vi "SystemNSOM.vi"() -> ()   [LabVIEW 2018]
uses:
  <vilib>/Math Plots/3D Math Plots/3D Mesh/3D Mesh XCtrl/3D Mesh.xctl
  <vilib>/Math Plots/3D Math Plots/3D Mesh/3D Mesh Datatype/3D Mesh Datatype.lvclass
  <vilib>/Math Plots/3D Math Plots/3D Mesh/3D Mesh Datatype/Public/Plot Helper (Vector).vi
panel:
  in  "thr. Ang":dbl
  out "diff Ph":dbl=9.8
  out "err R":dbl=0.1226366888094022
  in  "NUMERO DE MED.":i32=1 min=1 max=10
  in  "ControlP":T1
  in  "thr":dbl=0.1
  out "th":bool
  out "Mult inic.":dbl
  out "lock in inic.":dbl
  out "A":dbl
  in  "Nombre imagenes":string
  in  "Nombre del  Archivo":string="test_0510_01"
  in  "Atributos":T2
  in  "stop":bool
  in  "tipo":enum32{"medicion", "visualizar"}(tab)
  in  "Medir  offset":bool
  out "Z nano":dbl=15415.0
  out "Y nano":dbl=2000.0
  out "X nano":dbl=88000.0
  out "Multimetro":dbl=-0.0012043666666666666
  out "Lock in":dbl=-0.0011005000000000001
  out "X":dbl
  in  "lockinMult":T3={"Num.Lect"=3, "Delay (ms)"=1000, "usar multimetro"=TRUE, "Num. Med"=3} {"Delay (ms)" min=100; "Num.Lect" min=1}
  out "AFM":refnum<class "3D Plot Datatype.lvclass">[](xcontrol)
  in  "tipoMed":enum16{"R", "AFM", "DRL", "DRC"}(ring)
  in  "movXYZ":T4={"Inicio x"=0.0, "Inicio y"=0.0, "fin x"=88000.0, "fin y "=2000.0, "paso"=2000.0, "selector"=FALSE}
  out "Lockin":refnum<class "3D Plot Datatype.lvclass">[](xcontrol)
  in  "Inicio":bool
  out "Y":dbl
  out "Z":dbl
  out "multimetro":refnum<class "3D Plot Datatype.lvclass">[](xcontrol)
  in  "Distancia de medicion":dbl=9.0
  out "Amplitud":dbl[](graph)=[0.0001737, 0.0001907, 0.0001951, 0.0001957, 0.0001958, 0.0001961, 0.0001961, 0.000196, 0.0001957, 0.0001957, 0.000196, 0.000196, 0.0001958, 0.000196, 0.000196, 0.0001958, 0.0001957, 0.0001957, 0.000196, 0.0001963, 0.0001963, 0.0001966, 0.0001966, 0.0001963, 0.0001965, 0.0001967, 0.0001966, 0.0001966, 0.0001966, 0.0001968, 0.000197, 0.000197, 0.000197, 0.0001968, 0.0001967, 0.0001967, 0.0001966, 0.0001966, 0.0001962, 0.000196, 0.0001961, 0.0001963, 0.0001962, 0.0001962, 0.0001962, 0.0001963, 0.0001965, 0.0001963, 0.0001962, 0.0001961, 0.0001958, 0.0001958, 0.0001958, 0.0001957, 0.0001955, 0.0001955, 0.000196, 0.0001961, 0.0001958, 0.0001956, 0.000196, 0.0001958, 0.0001958, 0.000196, 0.0001958, 0.000196, 0.0001958, 0.0001958, 0.0001958, 0.0001956, 0.0001952, 0.0001952, 0.0001956, 0.0001956, 0.0001957, 0.0001956, 0.0001955, 0.0001958, 0.0001958, 0.0001961, 0.0001962, 0.0001962, 0.0001963, 0.0001966, 0.0001965, 0.0001966, 0.0001966, 0.0001968, 0.0001968, 0.0001966, 0.0001961, 0.0001962, 0.0001965, 0.0001967, 0.0001963, 0.0001961, 0.0001958, 0.0001963, 0.0001966, 0.0001965, 0.0001963, 0.0001961, 0.0001961, 0.0001966, 0.0001968, 0.0001967, 0.0001963, 0.0001961, 0.0001961, 0.0001961, 0.0001958, 0.0001957, 0.0001956, 0.0001957, 0.0001955, 0.0001956, 0.0001958, 0.0001952, 0.0001958, 0.0001958, 0.0001955, 0.0001955, 0.0001955, 0.0001961, 0.0001963, 0.0001965, 0.0001962, 0.000196, 0.0001963, 0.0001966, 0.0001966, 0.0001966, 0.0001963, 0.0001963, 0.0001966, 0.0001966, 0.0001966, 0.0001965, 0.0001963, 0.0001966, 0.0001967, 0.0001968, 0.0001967, 0.0001966, 0.0001966, 0.0001967, 0.0001966, 0.0001965, 0.0001963, 0.0001967, 0.0001963, 0.0001961, 0.0001956, 0.0001956, 0.0001956, 0.0001956, 0.0001955, 0.0001952, 0.0001952, 0.0001952, 0.0001955, 0.0001957, 0.0001956, 0.0001956, 0.0001956, 0.0001957, 0.0001958, 0.0001958, 0.0001956, 0.0001955, 0.0001956, 0.0001958, 0.0001957, 0.0001956, 0.0001956, 0.0001956, 0.0001958, 0.0001957, 0.0001955, 0.0001956, 0.000196, 0.0001958, 0.0001961, 0.000196, 0.000196, 0.0001958, 0.0001965, 0.0001963, 0.0001966, 0.0001965, 0.0001965, 0.0001965, 0.0001963, 0.0001963, 0.0001961, 0.0001961, 0.0001966, 0.0001966, 0.0001966, 0.0001965, 0.0001958, 0.000196, 0.0001962, 0.0001962, 0.0001965, 0.0001962, 0.0001963, 0.0001965, 0.0001963, 0.0001965, 0.0001961, 0.0001961, 0.0001961, 0.0001961, 0.0001962, 0.000196, 0.0001956, 0.0001961, 0.0001961, 0.0001958, 0.0001956, 0.0001953, 0.0001953, 0.0001956, 0.0001956, 0.0001953, 0.0001953, 0.0001955, 0.0001956, 0.0001955, 0.0001953, 0.0001952, 0.0001952, 0.0001957, 0.0001958, 0.0001958, 0.0001958, 0.0001958, 0.0001958, 0.0001958, 0.0001956, 0.0001955, 0.0001957, 0.000196, 0.0001961, 0.0001958, 0.0001957, 0.0001957, 0.0001958, 0.0001961, 0.0001961, 0.0001961, 0.0001958, 0.0001958, 0.0001961, 0.0001965, 0.0001963, 0.0001965, 0.0001965, 0.0001965, 0.0001962, 0.0001963, 0.0001963, 0.0001961, 0.0001961, 0.0001958, 0.0001958, 0.000196, 0.0001958, 0.0001955, 0.0001956, 0.0001958, 0.0001956, 0.0001955, 0.0001957, 0.0001958, 0.0001958, 0.0001958, 0.0001956, 0.0001953, 0.0001953, 0.0001955, 0.0001953, 0.000195, 0.0001947, 0.0001948, 0.0001951, 0.0001951, 0.000195, 0.0001946, 0.0001948, 0.0001948, 0.0001952, 0.000195, 0.000195, 0.0001953, 0.0001956, 0.0001956, 0.0001958, 0.0001958, 0.0001961, 0.0001961, 0.000196, 0.0001958, 0.000196, 0.0001962, 0.0001965, 0.0001961, 0.000196, 0.0001955, 0.0001975, 0.0001981, 0.0001973, 0.0001966, 0.0001957, 0.0001953, 0.0001948, 0.0001946, 0.0001942, 0.0001933, 0.0001905, 0.0001845, 0.0001812, 0.0001717]
  out "Fase":dbl[](graph)=[1.35, -1.7, -2.3, -2.4, -2.4, -2.4, -2.35, -2.4, -2.4, -2.45, -2.45, -2.45, -2.45, -2.4, -2.4, -2.4, -2.4, -2.4, -2.45, -2.4, -2.4, -2.4, -2.4, -2.4, -2.45, -2.45, -2.45, -2.45, -2.5, -2.45, -2.4, -2.45, -2.4, -2.4, -2.4, -2.4, -2.45, -2.4, -2.45, -2.5, -2.5, -2.5, -2.45, -2.45, -2.5, -2.5, -2.45, -2.45, -2.45, -2.45, -2.45, -2.45, -2.45, -2.45, -2.5, -2.5, -2.45, -2.45, -2.45, -2.5, -2.5, -2.45, -2.4, -2.4, -2.4, -2.4, -2.45, -2.45, -2.45, -2.45, -2.5, -2.45, -2.45, -2.45, -2.4, -2.45, -2.5, -2.45, -2.5, -2.5, -2.55, -2.45, -2.45, -2.45, -2.45, -2.45, -2.45, -2.45, -2.45, -2.4, -2.45, -2.45, -2.45, -2.45, -2.45, -2.55, -2.6, -2.5, -2.5, -2.45, -2.5, -2.55, -2.6, -2.55, -2.45, -2.45, -2.45, -2.5, -2.5, -2.55, -2.45, -2.45, -2.45, -2.55, -2.5, -2.45, -2.55, -2.55, -2.5, -2.45, -2.5, -2.5, -2.5, -2.5, -2.45, -2.45, -2.45, -2.55, -2.55, -2.5, -2.5, -2.5, -2.55, -2.55, -2.5, -2.5, -2.5, -2.55, -2.55, -2.55, -2.55, -2.55, -2.55, -2.45, -2.55, -2.5, -2.5, -2.45, -2.5, -2.55, -2.5, -2.5, -2.55, -2.55, -2.55, -2.55, -2.55, -2.6, -2.65, -2.6, -2.55, -2.45, -2.45, -2.5, -2.55, -2.55, -2.55, -2.55, -2.5, -2.6, -2.55, -2.65, -2.55, -2.55, -2.55, -2.5, -2.6, -2.55, -2.55, -2.6, -2.6, -2.6, -2.55, -2.6, -2.6, -2.6, -2.65, -2.6, -2.55, -2.55, -2.55, -2.55, -2.5, -2.55, -2.6, -2.65, -2.7, -2.65, -2.65, -2.65, -2.7, -2.7, -2.6, -2.65, -2.65, -2.65, -2.6, -2.6, -2.55, -2.65, -2.65, -2.6, -2.6, -2.55, -2.55, -2.55, -2.6, -2.6, -2.55, -2.6, -2.6, -2.65, -2.6, -2.65, -2.55, -2.6, -2.55, -2.55, -2.6, -2.6, -2.6, -2.65, -2.6, -2.6, -2.6, -2.6, -2.65, -2.6, -2.6, -2.5, -2.55, -2.6, -2.7, -2.65, -2.6, -2.65, -2.7, -2.7, -2.7, -2.6, -2.55, -2.55, -2.6, -2.65, -2.6, -2.55, -2.6, -2.7, -2.7, -2.65, -2.6, -2.6, -2.6, -2.6, -2.55, -2.6, -2.65, -2.6, -2.65, -2.55, -2.5, -2.5, -2.55, -2.55, -2.6, -2.6, -2.65, -2.65, -2.6, -2.65, -2.65, -2.65, -2.65, -2.7, -2.65, -2.6, -2.6, -2.55, -2.55, -2.55, -2.65, -2.6, -2.65, -2.6, -2.65, -2.65, -2.65, -2.65, -2.65, -2.65, -2.6, -2.6, -2.6, -2.65, -2.65, -2.7, -2.65, -2.6, -2.55, 1.85, 14.25, 17.75, 19.65, 21.45, 22.75, 23.6, 24.45, 25.2, 25.05, 23.35, 15.35, 3.05, 0.4, 7.4]
  in  "Tipo Stop":enum16{"Amplitud", "Fase"}(ring)
  in  "nanoREc":bool
  in  "Ajuste":bool
  in  "camara":bool
  # "Lock in"
  # "Multimetro"
  # "Parámetros de barrido"
  # "micras"
  # "nanometros"
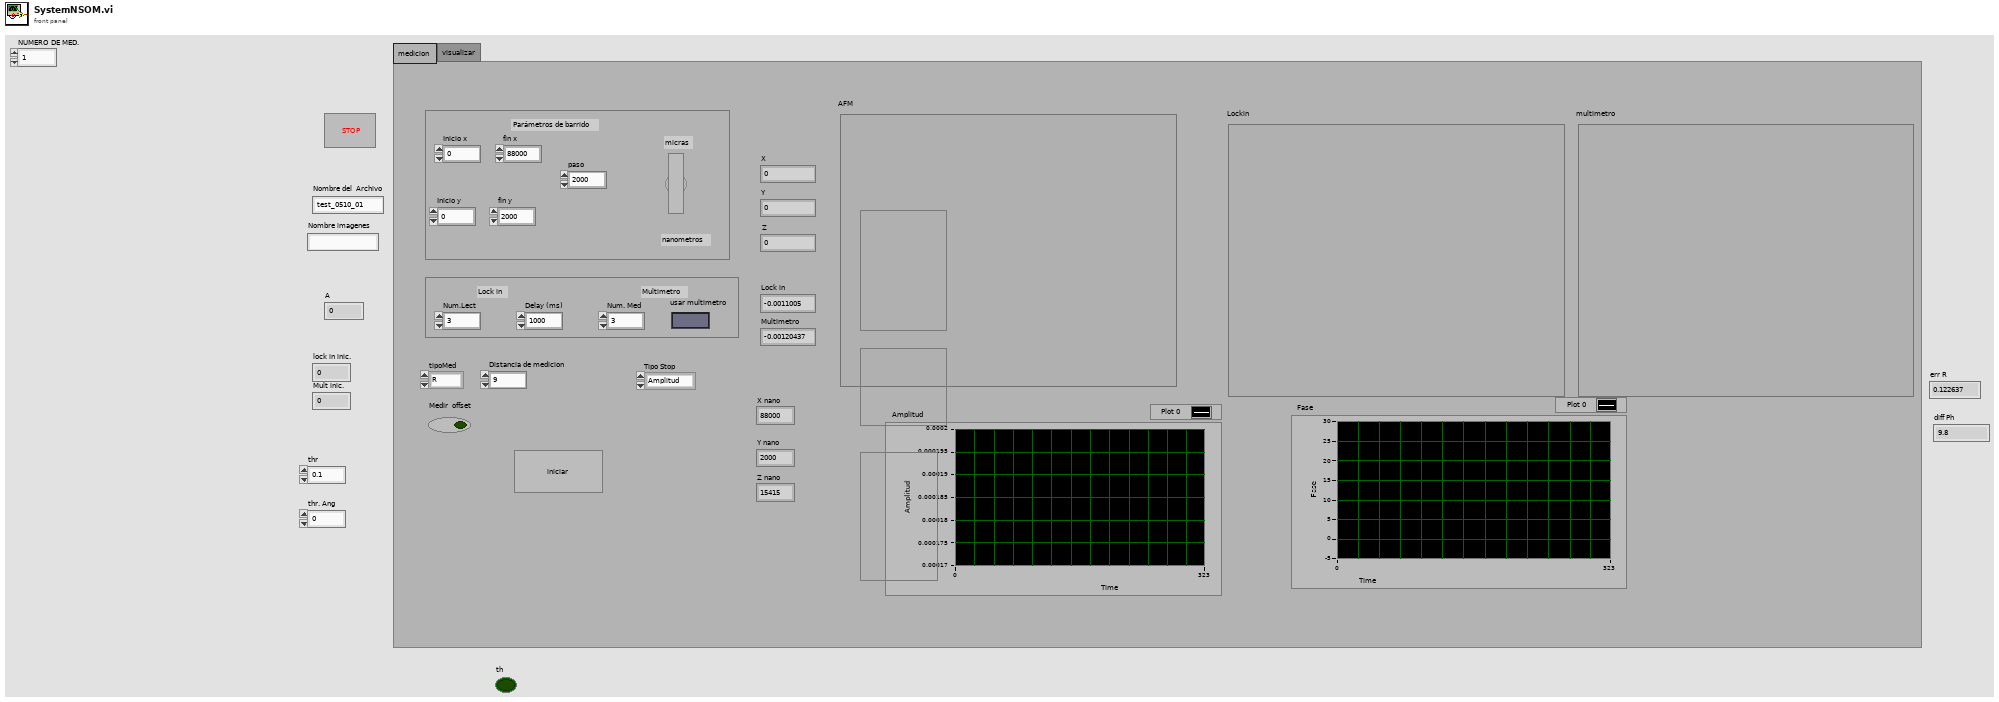
[diagram p1: front panel]
types:
  T1 = cluster{"posicion":dbl, "Amplitud":dbl[], "Fase":dbl[], "Err A":dbl, "Dif Ph":dbl, "Inic. A":dbl, "Inic. Ph":dbl}
  T2 = cluster{"Inicio X":dbl, "Inicio Y":dbl, "fin X ":dbl, "paso":dbl, "fin Y ":dbl, "Unidades":string, "Tipo":string}
  T3 = cluster{"Num.Lect":i32, "Delay (ms)":i32, "usar multimetro":bool, "Num. Med":i32}
  T4 = cluster{"Inicio x":dbl, "Inicio y":dbl, "fin x":dbl, "fin y ":dbl, "paso":dbl, "selector":bool}
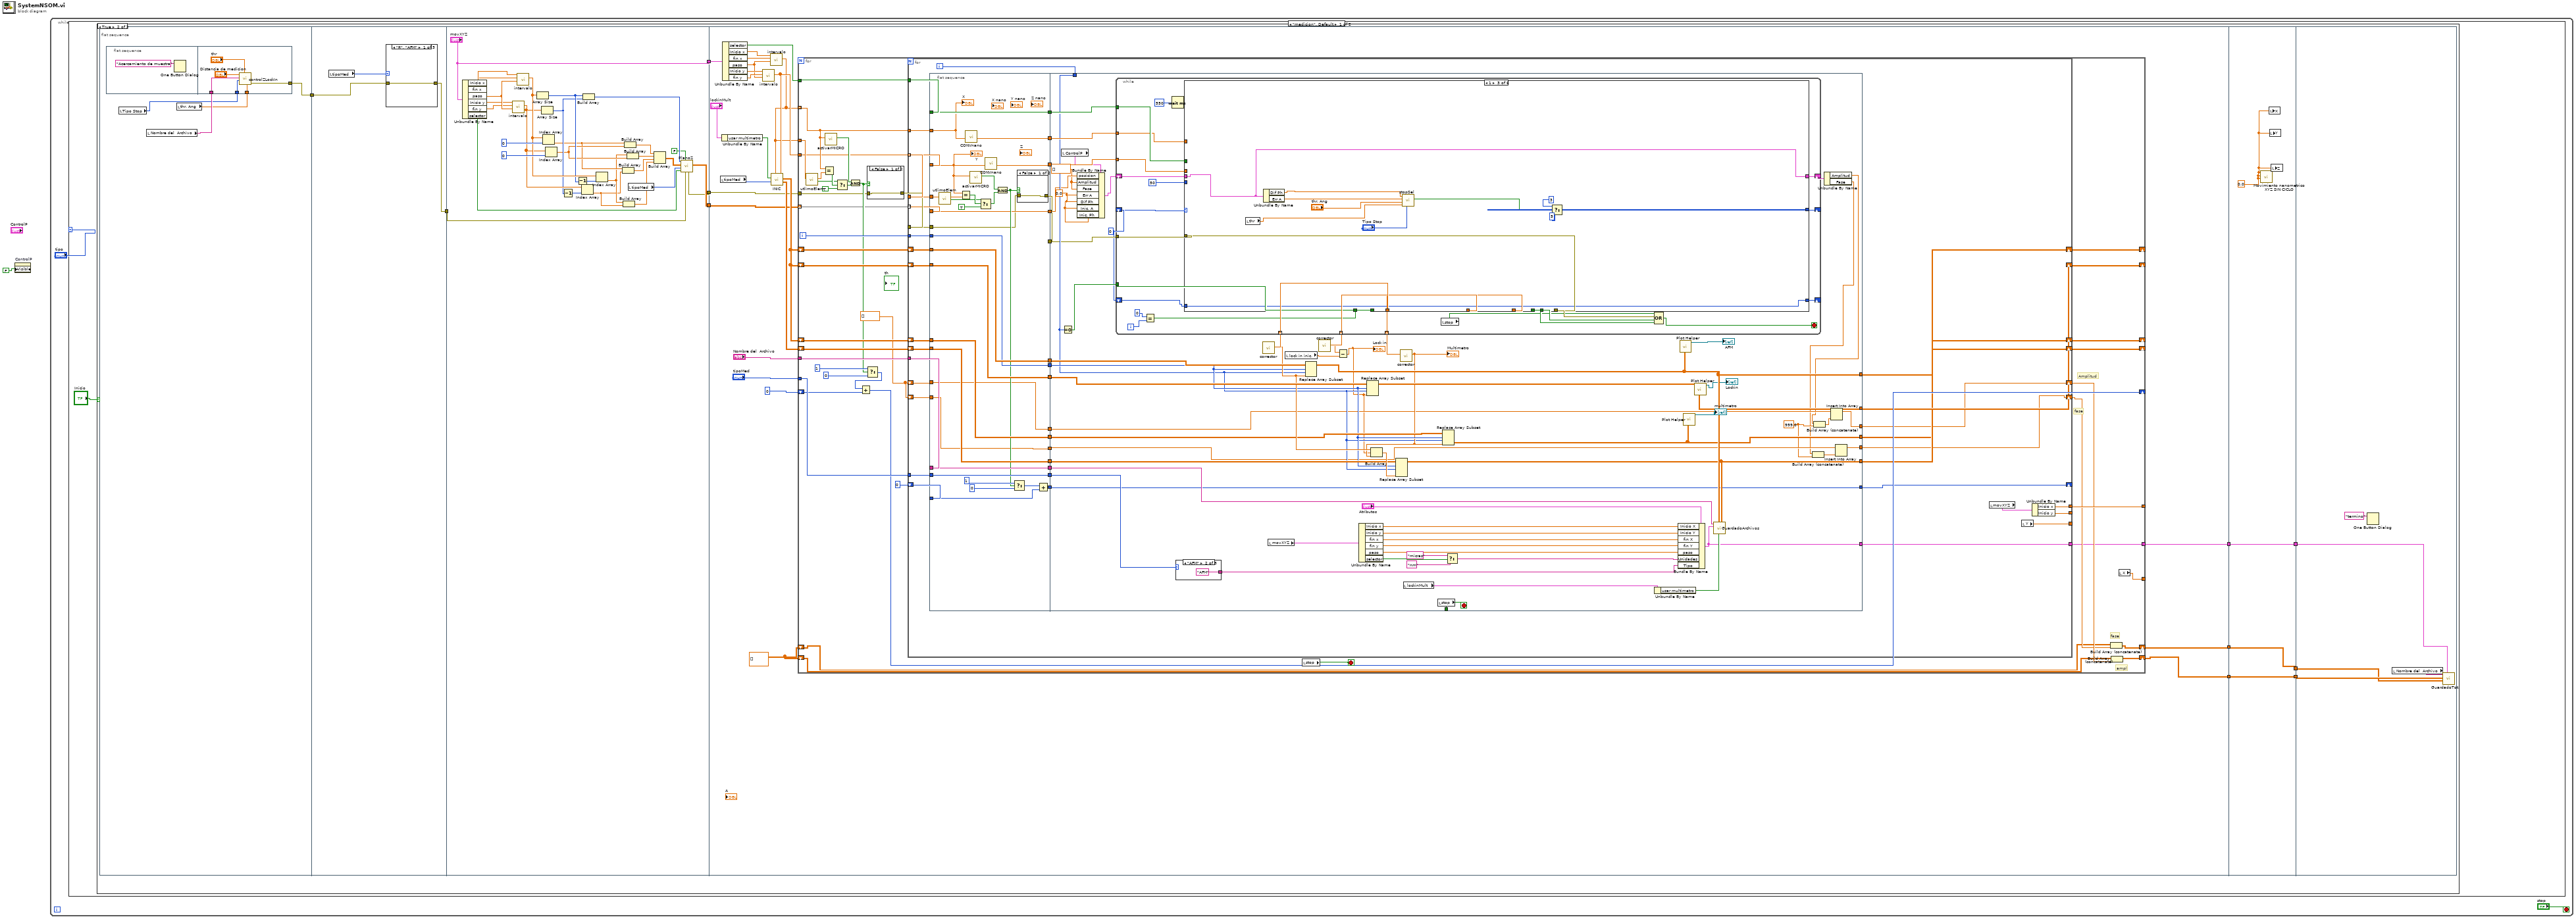
[diagram p0: block diagram]
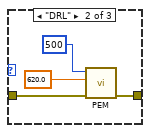
[diagram p3: hidden frame]
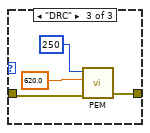
[diagram p4: hidden frame]
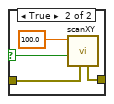
[diagram p5: hidden frame]
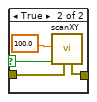
[diagram p6: hidden frame]
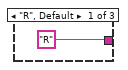
[diagram p7: hidden frame]
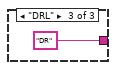
[diagram p8: hidden frame]
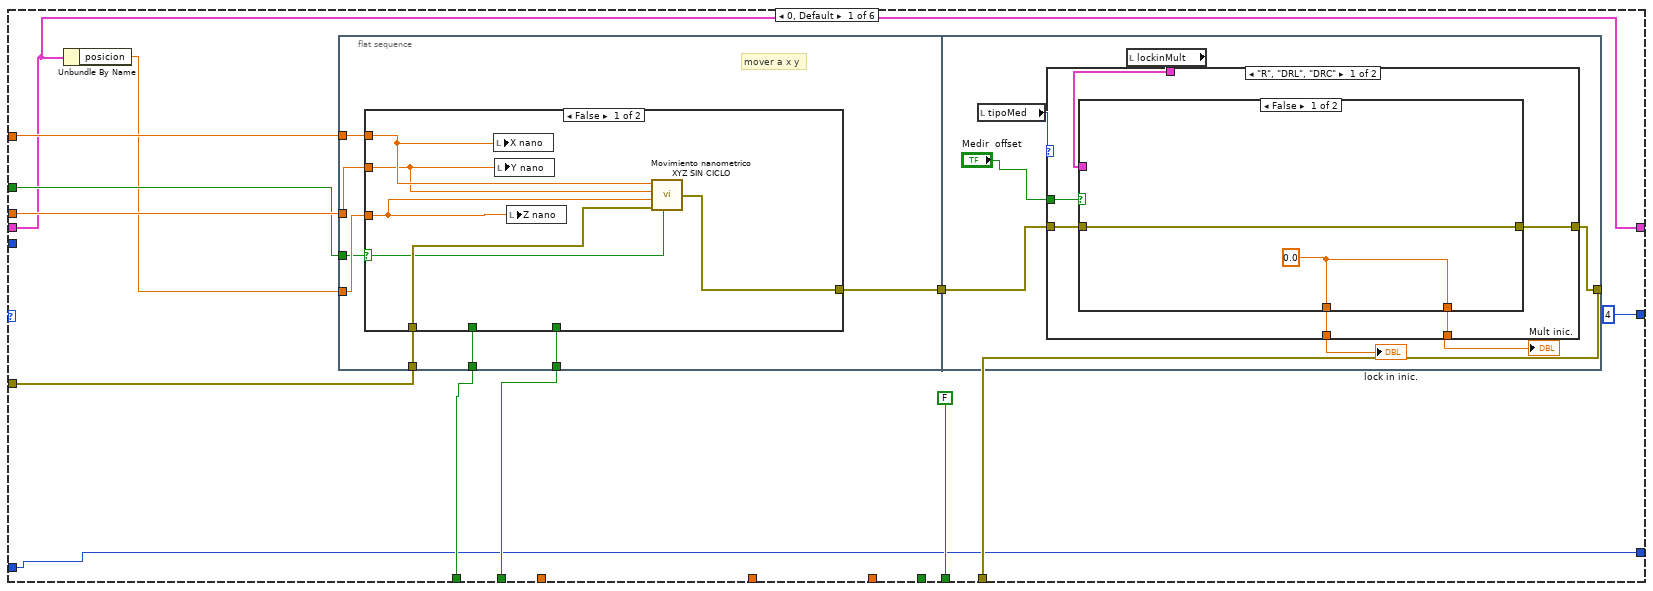
[diagram p9: hidden frame]
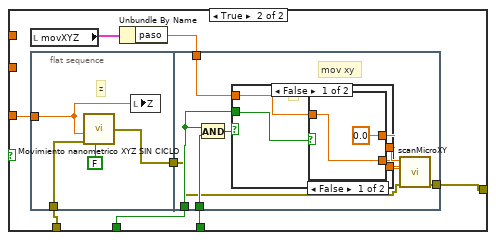
[diagram p10: hidden frame]
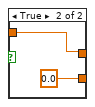
[diagram p11: hidden frame]
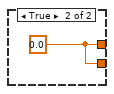
[diagram p12: hidden frame]
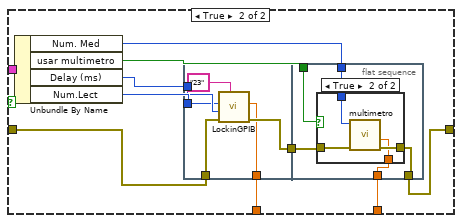
[diagram p13: hidden frame]
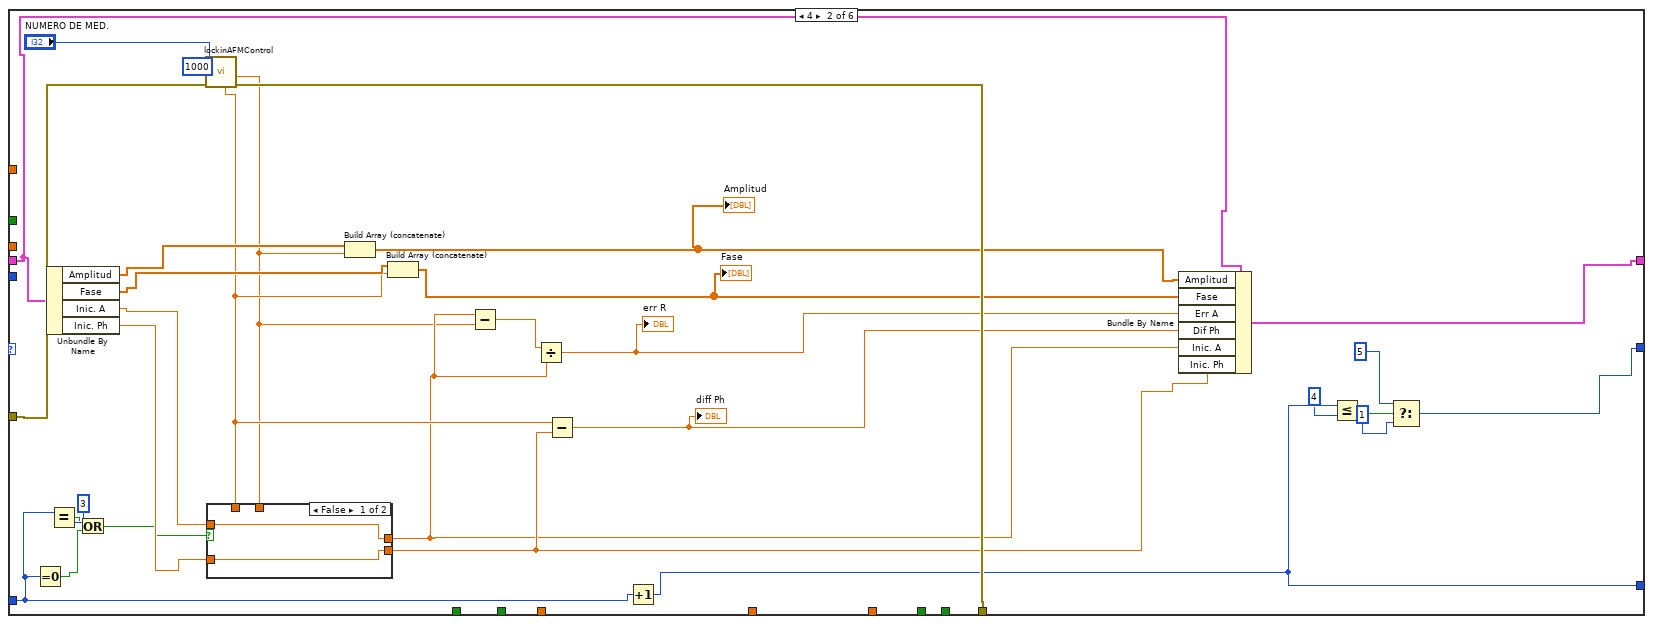
[diagram p16: hidden frame]
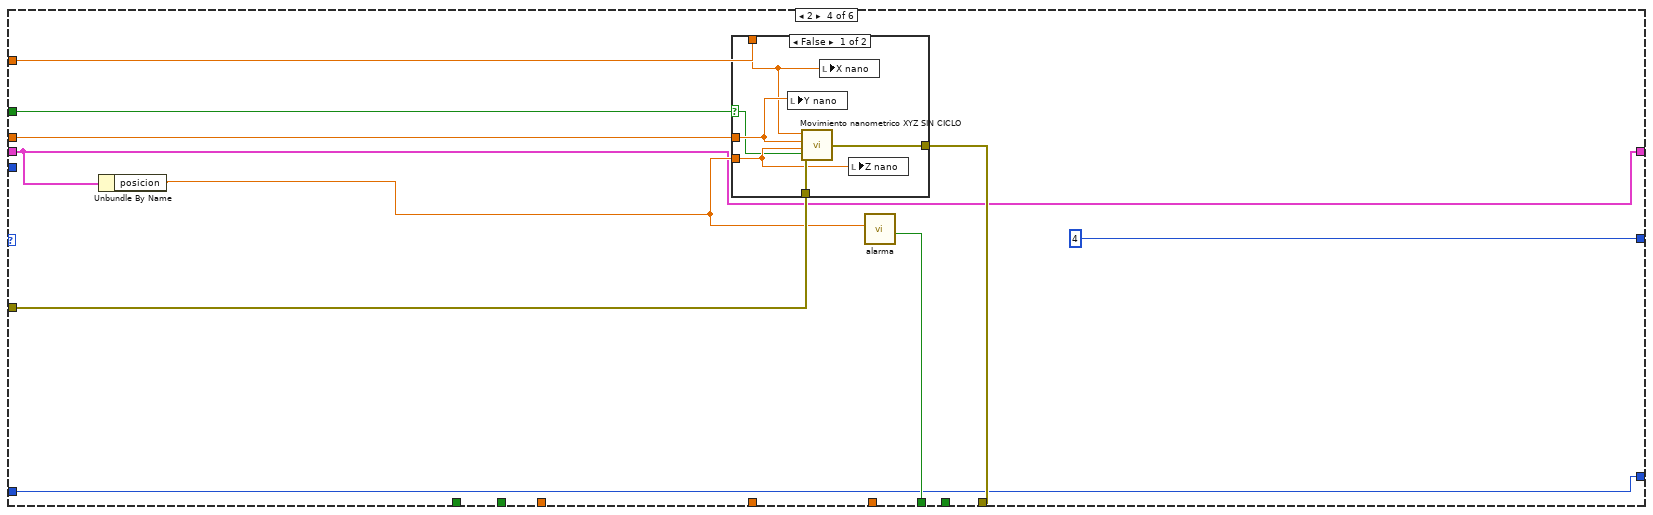
[diagram p18: hidden frame]
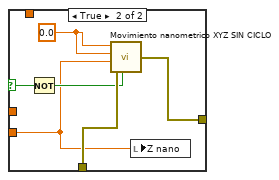
[diagram p19: hidden frame]
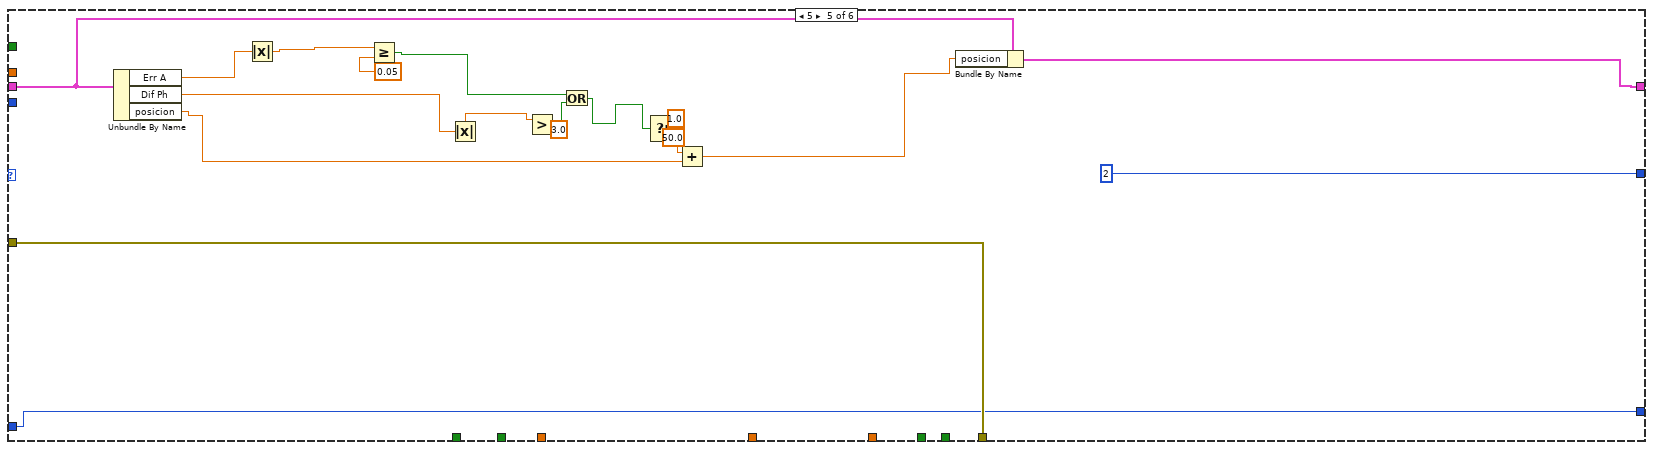
[diagram p20: hidden frame]
diagram:
  n1 = property on="ControlP" class="Clust (strict)"("Visible"=FALSE) -> ()  [unwired: 2 in, 2 out]
  n2 = while {
    stop <- "stop" stop-if-true
    n3 = case shown="\"medicion\", Default" "tipo" {
      frame "medicion", Default {
        n4 = case shown="True" "Inicio" {
          frame False {
          }
          frame True {
            n5 = flat-sequence {
              tunnel: [w19] -> w11
              tunnel: [w28] -> w12
              tunnel: w11 -> [w27]
              tunnel: ["movXYZ"] -> w15
              tunnel: [w44] -> w14
              tunnel: [w42] -> w13
              tunnel: w12 -> [w41]
              tunnel: w15 -> [w76]
              tunnel: w14 -> [w75]
              tunnel: w13 -> [w72]
              tunnel: [w73] -> w10
              tunnel: [w70] -> w7
              tunnel: [w69] -> w5
              tunnel: w10 -> [w571]
              tunnel: [w571] -> w9
              tunnel: [w570] -> w8
              tunnel: w7 -> [w570]
              tunnel: [w569] -> w6
              tunnel: w5 -> [w569]
              tunnel: w9 -> [w576]
              tunnel: w8 -> [w575]
              tunnel: w6 -> [w573]
              frame #0 {
                n6 = flat-sequence {
                  tunnel: [w25] -> w19
                  tunnel: w18 -> [w24]
                  tunnel: w17 -> [w22]
                  tunnel: w16 -> [w21]
                  frame #0 {
                    n7 = One Button Dialog(message="Acercamiento de muestra") -> ()  [unwired: 1 in, 1 out]
                  }
                  frame #1 {
                    n8 = call "controlZLockIn.vi"("thrAng"=w22, "thr"="thr", "Tipo"=w21, "name"=w24, "Distancia de medicion"="Distancia de medicion") -> ("error out"=w25:errorcluster)  [unwired: 3 in, 3 out]
                  }
                }
                n9 = local read "Tipo Stop"() -> (w16:enum16{"Amplitud", "Fase"})
                n10 = local read "Nombre del  Archivo"() -> (w18:string)
                n11 = local read "thr. Ang"() -> (w17:dbl)
              }
              frame #1 {
                n12 = local read "tipoMed"() -> (w29:enum16{"R", "AFM", "DRL", "DRC"})
                n13 = case shown="\"R\", \"AFM\"" w29 {
                  tunnel: [w30 w32 w36] -> w28
                  tunnel: w27 -> [w30 w31 w35]
                  frame "R", "AFM" {
                  }
                  frame "DRL" {
                    n14 = call "PEM.vi"("error in (no error)"=w31, "Longitud de Onda"=620.0, "Retardo"=500) -> ("error out"=w32:errorcluster)  [unwired: 6 in, 2 out]
                  }
                  frame "DRC" {
                    n15 = call "PEM.vi"("error in (no error)"=w35, "Longitud de Onda"=620.0, "Retardo"=250) -> ("error out"=w36:errorcluster)  [unwired: 6 in, 2 out]
                  }
                }
              }
              frame #2 {
                n16 = Unbundle By Name("movXYZ") -> ("Inicio x"=w67:dbl, "fin x"=w66:dbl, "paso"=w65:dbl, "Inicio y"=w64:dbl, "fin y"=w63:dbl, "selector"=w40:bool)
                n17 = call "intervalo.vi"("incremento"=w65, "fin"=w63, "inicio"=w64) -> ("Array"=w58:dbl[])  [unwired: 8 in]
                n18 = call "intervalo.vi"("incremento"=w65, "fin"=w66, "inicio"=w67) -> ("Array"=w59:dbl[])  [unwired: 8 in]
                n19 = Array Size(array=w59) -> (size(s)=w57:i32)
                n20 = Array Size(array=w58) -> (size(s)=w55:i32)
                n21 = Index Array(array=w59, index=0) -> (element=w52:dbl)
                n22 = Index Array(array=w58, index=0) -> (element=w53:dbl)
                n23 = Decrement(x=w55) -> (x-1=w54:i32)
                n24 = Decrement(x=w57) -> (x-1=w56:i32)
                n25 = Index Array(array=w58, index=w54) -> (element=w50:dbl)
                n26 = Build Array(w57, w55) -> (w62:i32[])
                n27 = Index Array(array=w59, index=w56) -> (element=w51:dbl)
                n28 = Build Array(w52, w50) -> (w47:dbl[])
                n29 = Build Array(w51, w50) -> (w46:dbl[])
                n30 = Build Array(w52, w53) -> (w49:dbl[])
                n31 = Build Array(w51, w53) -> (w48:dbl[])
                n32 = local read "tipoMed"() -> (w43:enum16{"R", "AFM", "DRL", "DRC"})
                n33 = Build Array(w49, w48, w47, w46) -> (w45:dbl[][])
                n34 = call "PlanoZ.vi"("error in (no error)"=w41, "Pendiente"=FALSE, "tipo"=w40, "tipoMed"=w43, "MedicionesPuntos"=w45, "Tamaños"=w62) -> ("PosZ"=w44:dbl[][], "error out"=w42:errorcluster)  [unwired: 4 in]
              }
              frame #3 {
                w71 = dbl[][] []
                n35 = local read "tipoMed"() -> (w78:enum16{"R", "AFM", "DRL", "DRC"})
                n36 = Unbundle By Name("lockinMult") -> ("usar multimetro"=w81:bool)
                n37 = Unbundle By Name(w76) -> ("selector"=w86:bool, "Inicio x"=w90:dbl, "fin x"=w91:dbl, "paso"=w87:dbl, "Inicio y"=w89:dbl, "fin y"=w88:dbl)
                n38 = call "intervalo.vi"("incremento"=w87, "fin"=w88, "inicio"=w89) -> ("Array"=w85:dbl[])  [unwired: 8 in]
                n39 = call "intervalo.vi"("incremento"=w87, "fin"=w91, "inicio"=w90) -> ("Array"=w74:dbl[])  [unwired: 8 in]
                n40 = call "INIC.vi"("ArrY"=w85, "ArrX"=w74, "tipoMed"=w78, "mutl"=w81) -> ("ArrSal4"=w80:dbl[][][], "ArrSAL"=w79:dbl[][])  [unwired: 6 in]
                n41 = for {
                  tunnel: w74 -> [w109] mode=indexing
                  tunnel: w85 -> [w107]
                  tunnel: w86 -> [w133]
                  shift-right: [w131] -> _
                  shift-left: w79 -> [w132]
                  tunnel: "tipoMed" -> [w129]
                  tunnel: "Nombre del  Archivo" -> [w128]
                  shift-right: [w126] -> _
                  shift-left: w79 -> [w127]
                  shift-right: [w124] -> _
                  shift-left: w80 -> [w125]
                  shift-right: [w121] -> _
                  shift-left: w79 -> [w122]
                  shift-right: [w110] -> _
                  shift-left: 0 -> [w111]
                  tunnel: w74 -> [w108]
                  tunnel: w75 -> [w104] mode=indexing
                  tunnel: w72 -> [w102]
                  tunnel: [w101] -> _
                  tunnel: [w100] -> _
                  shift-right: [w99] -> w73
                  shift-left: w71 -> [w97]
                  shift-right: [w95] -> w70
                  shift-left: w71 -> [w93]
                  tunnel: [w92] -> w69
                  i -> [w130]
                  stop <- w123 stop-if-true
                  w96 = dbl[] []
                  # "ampl"
                  # "fase"
                  # "fase"
                  # "Amplitud"
                  n42 = call "utlimoElem.vi"("Elementos"=w108) -> ("x = 0?"=w118:bool, "element"=w120:dbl)  [unwired: 9 in]
                  n43 = Equal?(x=w109, y=w120) -> (x = y?=w119:bool)
                  n44 = call "activarMICRO.vi"("valor"=w109) -> ("Indicador"=w115:bool)  [unwired: 10 in]
                  n45 = Select(t=w118, s=w119, f=TRUE) -> (s? t:f=w116:bool)
                  n46 = And(x=w115, y=w116) -> (x .and. y?=w105:bool)
                  n47 = case shown="False" w105 {
                    selector: w105 -> [_ w137]
                    tunnel: [w134 w136] -> w103
                    tunnel: w102 -> [w134 w135]
                    frame False {
                    }
                    frame True {
                      n48 = call "scanXY.vi"("Error In"=w135, "Activar movimiento en X"=w137, "Micras en X"=100.0) -> ("Error Out"=w136:errorcluster)  [unwired: 8 in]
                    }
                  }
                  n49 = Select(t=1, s=w105, f=0) -> (s? t:f=w114:i32)
                  n50 = Add(x=w114, y=w111) -> (x+y=w110:i32)
                  n51 = for {
                    tunnel: w109 -> [w181]
                    tunnel: w107 -> [w182] mode=indexing
                    tunnel: w133 -> [w183]
                    shift-right: [w179] -> w131
                    shift-left: w132 -> [w180]
                    tunnel: w130 -> [w170]
                    tunnel: w129 -> [w178]
                    tunnel: w128 -> [w177]
                    shift-right: [w174] -> w126
                    shift-left: w127 -> [w176]
                    shift-right: [w173] -> w124
                    shift-left: w125 -> [w175]
                    shift-right: [w168] -> w121
                    shift-left: w122 -> [w171]
                    tunnel: w107 -> [w167]
                    shift-right: [w165] -> _
                    shift-left: 0 -> [w166]
                    tunnel: w104 -> [w164] mode=indexing
                    tunnel: w103 -> [w163]
                    tunnel: [w162] -> _
                    tunnel: [w160] -> w101
                    tunnel: [w159] -> _
                    shift-right: [w157] -> w98
                    shift-left: w96 -> [w158]
                    shift-right: [w140] -> w94
                    shift-left: w96 -> [w141]
                    tunnel: [w139] -> w92
                    i -> [w169]
                    stop <- w172 stop-if-true
                    n52 = flat-sequence {
                      tunnel: w170 -> [w206]
                      tunnel: w171 -> [w207]
                      tunnel: w175 -> [w208]
                      tunnel: w176 -> [w209]
                      tunnel: w177 -> [w210]
                      tunnel: w178 -> [w211]
                      tunnel: w180 -> [w212]
                      tunnel: w181 -> [w193]
                      tunnel: w182 -> [w191]
                      tunnel: w183 -> [w213]
                      tunnel: [w213] -> w156
                      tunnel: [w190] -> w155
                      tunnel: [w192] -> w154
                      tunnel: [w212] -> w153
                      tunnel: [w211] -> w152
                      tunnel: [w210] -> w151
                      tunnel: [w209] -> w150
                      tunnel: [w208] -> w149
                      tunnel: [w207] -> w148
                      tunnel: [w206] -> w147
                      tunnel: w167 -> [w201]
                      tunnel: w166 -> [w195]
                      tunnel: [w194] -> w146
                      tunnel: [w188] -> w145
                      tunnel: w164 -> [w188]
                      tunnel: [w187] -> w144
                      tunnel: w163 -> [w186]
                      tunnel: w158 -> [w185]
                      tunnel: [w185] -> w143
                      tunnel: [w184] -> w142
                      tunnel: w141 -> [w184]
                      tunnel: [w271] -> w179
                      tunnel: [w255] -> w174
                      tunnel: [w254] -> w173
                      tunnel: [w251] -> w172
                      tunnel: w169 -> [w241]
                      tunnel: [w244] -> w168
                      tunnel: w156 -> [w280]
                      tunnel: w155 -> [w279]
                      tunnel: w154 -> [w278]
                      tunnel: w153 -> [w276]
                      tunnel: w152 -> [w262]
                      tunnel: w151 -> [w260]
                      tunnel: w150 -> [w258]
                      tunnel: w149 -> [w256]
                      tunnel: w148 -> [w247]
                      tunnel: w147 -> [w246]
                      tunnel: [w242] -> w165
                      tunnel: w146 -> [w242]
                      tunnel: w145 -> [w232]
                      tunnel: w144 -> [w240]
                      tunnel: w143 -> [w239]
                      tunnel: [w238] -> w157
                      tunnel: w142 -> [w226]
                      tunnel: [w225] -> w140
                      tunnel: [w224] -> w139
                      frame #0 {
                        n53 = call "utlimoElem.vi"("Elementos"=w201) -> ("x = 0?"=w200:bool, "element"=w205:dbl)  [unwired: 9 in]
                        n54 = Equal?(x=w191, y=w205) -> (x = y?=w204:bool)
                        n55 = call "CONVnano.vi"("vAL"=w193) -> ("NANO"=w192:dbl)  [unwired: 10 in]
                        n56 = call "activarMICRO.vi"("valor"=w191) -> ("Indicador"=w199:bool)  [unwired: 10 in]
                        n57 = Select(t=w200, s=w204, f=TRUE) -> (s? t:f=w202:bool)
                        n58 = call "CONVnano.vi"("vAL"=w191) -> ("NANO"=w190:dbl)  [unwired: 10 in]
                        n59 = And(x=w199, y=w202) -> (x .and. y?=w189:bool)
                        n60 = Select(t=1, s=w189, f=0) -> (s? t:f=w198:i32)
                        n61 = case shown="False" w189 {
                          selector: w189 -> [_ w217]
                          tunnel: [w214 w216] -> w187
                          tunnel: w186 -> [w214 w215]
                          frame False {
                          }
                          frame True {
                            n62 = call "scanXY.vi"("Error In"=w215, "Activar movimiento en Y"=w217, "Micras en Y"=100.0) -> ("Error Out"=w216:errorcluster)  [unwired: 8 in]
                          }
                        }
                        n63 = Add(x=w198, y=w195) -> (x+y=w194:i32)
                        "X" <- w193
                        "Y" <- w191
                      }
                      frame #1 {
                        w221 = 999.0
                        w229 = 0.0
                        w231 = dbl[] []
                        w228 = 0
                        n64 = local read "ControlP"() -> (w233:T1)
                        n65 = Equal To 0?(x=w241) -> (x = 0?=w234:bool)
                        n66 = Bundle By Name(cluster=w233, "posicion"=w232, "Amplitud"=w231, "Fase"=w231, "Err A"=w229, "Dif Ph"=w229, "Inic. A"=w229, "Inic. Ph"=w229) -> (w230:T1)
                        n67 = while {
                          shift-right: [w306] -> _
                          shift-left: w228 -> [w307]
                          tunnel: w280 -> [w305]
                          tunnel: w278 -> [w297]
                          tunnel: w279 -> [w296]
                          tunnel: [w304] -> w277 mode=indexing
                          tunnel: [w300] -> w259 mode=indexing
                          tunnel: [w295] -> w248 mode=indexing
                          tunnel: w234 -> [w291]
                          tunnel: w240 -> [w292]
                          shift-right: [w286] -> w227
                          shift-left: w230 -> [w287]
                          shift-right: [w284] -> _
                          shift-left: w228 -> [w285]
                          i -> [w290]
                          stop <- w303 stop-if-true
                          n68 = Equal?(x=0, y=w290) -> (x = y?=w289:bool)
                          n69 = Wait (ms)(milliseconds to wait=u32 550) -> ()  [unwired: 1 out]
                          n70 = case shown="1" w307 {
                            tunnel: [4 w410 w450 4 2 0] -> w306
                            tunnel: w305 -> [w314 _ _ w455 _ _]
                            tunnel: w292 -> [w320 w435 w449 w461 w491 w504]
                            tunnel: [w319 w432 w449 w459 w491 w503] -> w302
                            tunnel: w297 -> [w316 _ _ w456 _ _]
                            tunnel: w296 -> [w315 _ _ w457 _ _]
                            tunnel: [_ _ _ _ _ w507] -> w304
                            tunnel: [FALSE _ _ _ _ TRUE] -> w301
                            tunnel: [_ _ _ _ _ w502] -> w300
                            tunnel: 50 -> [_ _ _ _ _ _]
                            tunnel: [_ _ _ w458 _ _] -> w294
                            tunnel: [_ _ _ _ _ w500] -> w295
                            tunnel: w291 -> [w313 _ _ _ _ _]
                            tunnel: w289 -> [w312 _ _ _ _ _]
                            tunnel: w287 -> [w309 w429 w447 w453 w483 w495]
                            tunnel: [w309 w424 w447 w453 w481 w494] -> w286
                            tunnel: w285 -> [w308 w419 w446 w452 w480 w493]
                            tunnel: [w308 w414 w446 w452 w480 w493] -> w284
                            frame 0, Default {
                              n71 = Unbundle By Name(w309) -> ("posicion"=w310:dbl)
                              n72 = flat-sequence {
                                tunnel: w320 -> [w328]
                                tunnel: w316 -> [w326]
                                tunnel: w315 -> [w325]
                                tunnel: w310 -> [w324]
                                tunnel: w314 -> [w323]
                                tunnel: w313 -> [w322]
                                tunnel: w312 -> [w321]
                                tunnel: [w327] -> w311
                                tunnel: [w365] -> w319
                                tunnel: w311 -> [w370]
                                frame #0 {
                                # "mover a x y"
                                n73 = case shown="False" w323 {
                                selector: w323 -> [w329 _]
                                tunnel: w328 -> [w334 w339]
                                tunnel: [w333 w335] -> w327
                                tunnel: w326 -> [w332 _]
                                tunnel: w325 -> [w331 _]
                                tunnel: w324 -> [w330 w342]
                                tunnel: w322 -> [_ w336]
                                tunnel: w321 -> [_ w337]
                                frame False {
                                n74 = local write "X nano"(w332) -> ()
                                n75 = local write "Y nano"(w331) -> ()
                                n76 = local write "Z nano"(w330) -> ()
                                n77 = call "Movimiento nanometrico XYZ SIN CICLO.vi"("Micras"=w329, "Error In"=w334, "Movimiento en Z"=w330, "Movimiento en Y"=w331, "Movimiento en X"=w332) -> ("Error Out"=w333:errorcluster)  [unwired: 1 in]
                                }
                                frame True {
                                n78 = local read "movXYZ"() -> (w341:T4)
                                n79 = flat-sequence {
                                tunnel: w342 -> [w345]
                                tunnel: w339 -> [w344]
                                tunnel: [w343] -> w338
                                tunnel: w340 -> [w354]
                                tunnel: w338 -> [w348]
                                tunnel: w337 -> [w352]
                                tunnel: w336 -> [w351]
                                tunnel: [w347] -> w335
                                frame #0 {
                                # "z"
                                n80 = call "Movimiento nanometrico XYZ SIN CICLO.vi"("Micras"=FALSE, "Error In"=w344, "Movimiento en Z"=w345) -> ("Error Out"=w343:errorcluster)  [unwired: 3 in]
                                n81 = local write "Z"(w345) -> ()
                                }
                                frame #1 {
                                # "mov xy"
                                # "x"
                                n82 = And(x=w352, y=w351) -> (x .and. y?=w353:bool)
                                n83 = case shown="False" w353 {
                                tunnel: [w356 w363] -> w349
                                tunnel: [w355 w363] -> w350
                                tunnel: w354 -> [w357 _]
                                tunnel: w352 -> [w358 _]
                                frame False {
                                n84 = case shown="False" w358 {
                                tunnel: [0.0 ("paso") w362] -> w356
                                tunnel: w357 -> [w359 w362]
                                tunnel: [w359 0.0] -> w355
                                frame False {
                                }
                                frame True {
                                }
                                }
                                }
                                frame True {
                                w363 = 0.0
                                }
                                }
                                n85 = call "scanMicroXY.vi"("error in (no error)"=w348, "Mov Y"=w350, "Mov X"=w349) -> ("error out"=w347:errorcluster)  [unwired: 8 in]
                                }
                                }
                                n86 = Unbundle By Name(w341) -> ("paso"=w340:dbl)
                                }
                                }
                                }
                                frame #1 {
                                n87 = local read "tipoMed"() -> (w367:enum16{"R", "AFM", "DRL", "DRC"})
                                n88 = local read "lockinMult"() -> (w366:T3)
                                n89 = case shown="\"R\", \"DRL\", \"DRC\"" w367 {
                                tunnel: w366 -> [w376 _]
                                tunnel: [w375 w405] -> w365
                                tunnel: w370 -> [w374 w405]
                                tunnel: [w373 _] -> w368
                                tunnel: [w372 _] -> w369
                                tunnel: "Medir  offset" -> [w371 _]
                                frame "R", "DRL", "DRC" {
                                n90 = case shown="False" w371 {
                                tunnel: w376 -> [_ w387]
                                tunnel: [w378 w386] -> w375
                                tunnel: w374 -> [w378 w385]
                                tunnel: [w377 w380] -> w373
                                tunnel: [w377 w379] -> w372
                                frame False {
                                w377 = 0.0
                                }
                                frame True {
                                n91 = Unbundle By Name(w387) -> ("Num. Med"=w381:i32, "usar multimetro"=w382:bool, "Delay (ms)"=w384:i32, "Num.Lect"=w383:i32)
                                n92 = flat-sequence {
                                tunnel: w385 -> [w394]
                                tunnel: [w393] -> w388
                                tunnel: w384 -> [w391]
                                tunnel: w383 -> [w390]
                                tunnel: [w392] -> w379
                                tunnel: [w398] -> w386
                                tunnel: w388 -> [w399]
                                tunnel: [w397] -> w380
                                tunnel: w382 -> [w396]
                                tunnel: w381 -> [w395]
                                frame #0 {
                                n93 = call "LockinGPIB.vi"("P-LockIn"="23", "error in (no error)"=w394, "delay"=w391, "Num. Lect"=w390) -> ("error out"=w393:errorcluster, "LockIn"=w392:dbl)  [unwired: 6 in]
                                }
                                frame #1 {
                                n94 = case shown="True" w396 {
                                tunnel: w399 -> [w400 w404]
                                tunnel: [w400 w403] -> w398
                                tunnel: [_ w402] -> w397
                                tunnel: w395 -> [_ w401]
                                frame False {
                                }
                                frame True {
                                n95 = call "multimetro.vi"("error in (no error)"=w404, "mediciones"=w401) -> ("error out"=w403:errorcluster, "voltajeProm"=w402:dbl)  [unwired: 7 in, 1 out]
                                }
                                }
                                }
                                }
                                }
                                }
                                }
                                frame "AFM", Default {
                                }
                                }
                                "lock in inic." <- w369
                                "Mult inic." <- w368
                                }
                              }
                            }
                            frame 4 {
                              n96 = Equal To 0?(x=w419) -> (x = 0?=w416:bool)
                              n97 = Unbundle By Name(w429) -> ("Amplitud"=w428:dbl[], "Fase"=w427:dbl[], "Inic. A"=w430:dbl, "Inic. Ph"=w431:dbl)
                              n98 = Equal?(x=w419, y=3) -> (x = y?=w417:bool)
                              n99 = Or(x=w417, y=w416) -> (x .or. y?=w415:bool)
                              n100 = call "lockinAFMControl.vi"("error in"=w435, "NUMERO DE MED."="NUMERO DE MED.", "milliseconds to wait"=u32 1000) -> ("error out"=w432:errorcluster, "Prom. X"=w407:dbl, "Prom. Y"=w426:dbl)  [unwired: 4 in, 2 out]
                              n101 = case shown="False" w415 {
                                tunnel: w426 -> [_ w438]
                                tunnel: [w437 w439] -> w408
                                tunnel: w407 -> [_ w439]
                                tunnel: [w436 w438] -> w425
                                tunnel: w430 -> [w437 _]
                                tunnel: w431 -> [w436 _]
                                frame False {
                                }
                                frame True {
                                }
                              }
                              n102 = Build Array (concatenate)(w428, w407) -> (w423:dbl[])
                              "Amplitud" <- w423
                              n103 = Build Array (concatenate)(w427, w426) -> (w422:dbl[])
                              "Fase" <- w422
                              n104 = Subtract(x=w408, y=w407) -> (x-y=w406:dbl)
                              n105 = Divide(x=w406, y=w408) -> (x/y=w421:dbl)
                              "err R" <- w421
                              n106 = Subtract(x=w426, y=w425) -> (x-y=w420:dbl)
                              "diff Ph" <- w420
                              n107 = Increment(x=w419) -> (x+1=w414:i32)
                              n108 = Bundle By Name(cluster=w429, "Amplitud"=w423, "Fase"=w422, "Err A"=w421, "Dif Ph"=w420, "Inic. A"=w408, "Inic. Ph"=w425) -> (w424:T1)
                              n109 = Less Or Equal?(x=w414, y=4) -> (x <= y?=w412:bool)
                              n110 = Select(t=5, s=w412, f=1) -> (s? t:f=w410:i32)
                            }
                            frame 1 {
                              n111 = local read "thr"() -> (w443:dbl)
                              n112 = Unbundle By Name(w447) -> ("Dif Ph"=w440:dbl, "Err A"=w445:dbl)
                              n113 = call "stopSel.vi"("Tipo"="Tipo Stop", "thr"=w443, "thr. Ang"="thr. Ang", "Err.Amp"=w445, "DifFase"=w440) -> ("stop"=w442:bool)  [unwired: 6 in]
                              n114 = Select(t=3, s=w442, f=5) -> (s? t:f=w450:i32)
                            }
                            frame 2 {
                              n115 = Unbundle By Name(w453) -> ("posicion"=w454:dbl)
                              n116 = case shown="False" w455 {
                                selector: w455 -> [w462 w471]
                                tunnel: w461 -> [w467 w473]
                                tunnel: [w466 w472] -> w459
                                tunnel: w454 -> [w465 w468]
                                tunnel: w457 -> [w464 _]
                                tunnel: w456 -> [w463 _]
                                frame False {
                                n117 = local write "Y nano"(w464) -> ()
                                n118 = call "Movimiento nanometrico XYZ SIN CICLO.vi"("Micras"=w462, "Error In"=w467, "Movimiento en Z"=w465, "Movimiento en Y"=w464, "Movimiento en X"=w463) -> ("Error Out"=w466:errorcluster)  [unwired: 1 in]
                                n119 = local write "X nano"(w463) -> ()
                                n120 = local write "Z nano"(w465) -> ()
                                }
                                frame True {
                                w469 = 0.0
                                n121 = Not(x=w471) -> (.not. x?=w470:bool)
                                n122 = call "Movimiento nanometrico XYZ SIN CICLO.vi"("Micras"=w470, "Error In"=w473, "Movimiento en Z"=w468, "Movimiento en Y"=w469, "Movimiento en X"=w469) -> ("Error Out"=w472:errorcluster)  [unwired: 1 in]
                                n123 = local write "Z nano"(w468) -> ()
                                }
                              }
                              n124 = call "alarma.vi"("Valor"=w454) -> ("Boolean"=w458:bool)  [unwired: 10 in]
                            }
                            frame 5 {
                              n125 = Unbundle By Name(w483) -> ("Err A"=w475:dbl, "Dif Ph"=w486:dbl, "posicion"=w484:dbl)
                              n126 = Absolute Value(x=w475) -> (abs(x)=w474:dbl)
                              n127 = Greater Or Equal?(x=w474, y=0.05) -> (x >= y?=w478:bool)
                              n128 = Absolute Value(x=w486) -> (abs(x)=w487:dbl)
                              n129 = Greater?(x=w487, y=3.0) -> (0:w477:bool)
                              n130 = Or(x=w478, y=w477) -> (x .or. y?=w476:bool)
                              n131 = Select(t=1.0, s=w476, f=50.0) -> (s? t:f=w485:dbl)
                              n132 = Add(x=w485, y=w484) -> (x+y=w482:dbl)
                              n133 = Bundle By Name(cluster=w483, "posicion"=w482) -> (w481:T1)
                            }
                            frame 3 {
                              n134 = Unbundle By Name(w495) -> ("posicion"=w497:dbl)
                              n135 = local read "tipoMed"() -> (w508:enum16{"R", "AFM", "DRL", "DRC"})
                              n136 = local read "lockinMult"() -> (w501:T3)
                              n137 = case shown="\"R\", Default" w508 {
                                tunnel: [w513 w540 w546] -> w507
                                tunnel: w497 -> [w513 w540 w546]
                                tunnel: [0.0 0.0 0.0] -> w496
                                tunnel: w504 -> [w521 w538 w552]
                                tunnel: [w520 w538 w553] -> w503
                                tunnel: [w514 _ w545] -> w502
                                tunnel: w501 -> [w518 _ w550]
                                tunnel: [w515 _ w544] -> w500
                                tunnel: [TRUE w537 TRUE] -> w499
                                tunnel: [w510 w537 w541] -> w498
                                frame "R", Default {
                                n138 = Unbundle By Name(w518) -> ("Num. Med"=w517:i32, "usar multimetro"=w510:bool, "Num.Lect"=w509:i32, "Delay (ms)"=w516:i32)
                                n139 = flat-sequence {
                                tunnel: w521 -> [w526]
                                tunnel: [w524] -> w514
                                tunnel: [w525] -> w519
                                tunnel: w516 -> [w523]
                                tunnel: w509 -> [w522]
                                tunnel: [w530] -> w520
                                tunnel: w519 -> [w531]
                                tunnel: [w529] -> w515
                                tunnel: w510 -> [w528]
                                tunnel: w517 -> [w527]
                                frame #0 {
                                n140 = call "LockinGPIB.vi"("error in (no error)"=w526, "delay"=w523, "Num. Lect"=w522) -> ("error out"=w525:errorcluster, "LockIn"=w524:dbl)  [unwired: 7 in]
                                }
                                frame #1 {
                                n141 = case shown="True" w528 {
                                tunnel: w531 -> [w532 w536]
                                tunnel: [w532 w535] -> w530
                                tunnel: [_ w534] -> w529
                                tunnel: w527 -> [_ w533]
                                frame False {
                                }
                                frame True {
                                n142 = call "multimetro.vi"("error in (no error)"=w536, "mediciones"=w533) -> ("error out"=w535:errorcluster, "voltajeProm"=w534:dbl)  [unwired: 7 in, 1 out]
                                }
                                }
                                }
                                }
                                }
                                frame "AFM" {
                                w537 = FALSE
                                }
                                frame "DRL", "DRC" {
                                n143 = Unbundle By Name(w550) -> ("Num. Med"=w549:i32, "usar multimetro"=w541:bool, "Delay (ms)"=w548:i32, "Num.Lect"=w547:i32)
                                n144 = flat-sequence {
                                tunnel: w552 -> [w557]
                                tunnel: [w558] -> w551
                                tunnel: [w556] -> w545
                                tunnel: w547 -> [w555]
                                tunnel: w548 -> [w554]
                                tunnel: [w562] -> w553
                                tunnel: w551 -> [w563]
                                tunnel: [w561] -> w544
                                tunnel: w549 -> [w560]
                                tunnel: w541 -> [w559]
                                frame #0 {
                                # "lockin"
                                n145 = call "LockinGPIB.vi"("error in (no error)"=w557, "delay"=w554, "Num. Lect"=w555) -> ("error out"=w558:errorcluster, "LockIn"=w556:dbl)  [unwired: 7 in]
                                }
                                frame #1 {
                                n146 = case shown="True" w559 {
                                tunnel: w563 -> [w564 w568]
                                tunnel: [w564 w567] -> w562
                                tunnel: [_ w566] -> w561
                                tunnel: w560 -> [_ w565]
                                frame False {
                                }
                                frame True {
                                n147 = call "multimetro.vi"("error in (no error)"=w568, "mediciones"=w565) -> ("error out"=w567:errorcluster, "voltajeProm"=w566:dbl)  [unwired: 7 in, 1 out]
                                }
                                }
                                }
                                }
                                }
                              }
                              n148 = property on="Lockin" class="3D Mesh (strict)"("Visible"=w499) -> ()  [unwired: 2 in, 2 out]
                              n149 = property on="multimetro" class="3D Mesh (strict)"("Visible"=w498) -> ()  [unwired: 2 in, 2 out]
                              n150 = Bundle By Name(cluster=w495, "posicion"=w496) -> (w494:T1)
                            }
                          }
                          n151 = local read "stop"() -> (w293:bool)
                          n152 = Compound Arithmetic op=OR(w293, w302, w301, w294) -> (w303:bool)
                        }
                        n153 = case shown="\"AFM\"" w262 {
                          tunnel: ["R" "AFM" "DR"] -> w261
                          frame "R", Default {
                          }
                          frame "AFM" {
                          }
                          frame "DRL" {
                          }
                        }
                        n154 = call "corrector.vi"("Array"=w277) -> ("valor salida"=w250:dbl)  [unwired: 10 in]
                        n155 = local read "movXYZ"() -> (w274:T4)
                        n156 = local read "lock in inic."() -> (w235:dbl)
                        n157 = Replace Array Subset(array=w276, new element=w250, index (row)=w246, index (col)=w241) -> (w271:dbl[][])
                        n158 = call "corrector.vi"("Array"=w259) -> ("valor salida"=w237:dbl)  [unwired: 10 in]
                        n159 = Subtract(x=w237, y=w235) -> (x-y=w236:dbl)
                        "Lock in" <- w236
                        n160 = Unbundle By Name(w274) -> ("Inicio x"=w273:dbl, "Inicio y"=w270:dbl, "fin x"=w269:dbl, "fin y"=w268:dbl, "paso"=w267:dbl, "selector"=w266:bool)
                        n161 = Replace Array Subset(array=w258, new element=w236, index (row)=w246, index (col)=w241) -> (w255:dbl[][])
                        n162 = call "corrector.vi"("Array"=w248) -> ("valor salida"=w243:dbl)  [unwired: 10 in]
                        "Multimetro" <- w243
                        n163 = Build Array(w250, w236, w243) -> (w257:dbl[])
                        n164 = Replace Array Subset(array=w256, new element=w257, index (dim 0)=w246, index (dim 1)=w241) -> (w254:dbl[][][])  [unwired: 1 in]
                        n165 = local read "lockinMult"() -> (w253:T3)
                        n166 = local read "stop"() -> (w251:bool)
                        n167 = Replace Array Subset(array=w247, new element=w243, index (row)=w246, index (col)=w241) -> (w244:dbl[][])
                        n168 = Select(t="micras", s=w266, f="nm") -> (s? t:f=w264:string)
                        n169 = Unbundle By Name(w253) -> ("usar multimetro"=w252:bool)
                        n170 = Bundle By Name(cluster="Atributos", "Inicio X"=w273, "Inicio Y"=w270, "fin X"=w269, "fin Y"=w268, "paso"=w267, "Unidades"=w264, "Tipo"=w261) -> (w224:T2)
                        n171 = call-poly <vilib>:"Plot Helper.vi"("z matrix"=w271) -> ("3D Plot lvclass Array out"=→"AFM":refnum<class "3D Plot Datatype.lvclass">[])  [unwired: 5 in, 5 out]
                        n172 = call-poly <vilib>:"Plot Helper.vi"("z matrix"=w244) -> ("3D Plot lvclass Array out"=→"multimetro":refnum<class "3D Plot Datatype.lvclass">[])  [unwired: 5 in, 5 out]
                        n173 = call-poly <vilib>:"Plot Helper.vi"("z matrix"=w255) -> ("3D Plot lvclass Array out"=→"Lockin":refnum<class "3D Plot Datatype.lvclass">[])  [unwired: 5 in, 5 out]
                        n174 = call "GuardadoArchivos.vi"("DatosMULT"=w254, "Mult."=w252, "Datos"=w271, "Atributos"=w224, "Nombre"=w260) -> ()  [unwired: 6 in, 1 out]
                        n175 = Unbundle By Name(w227) -> ("Amplitud"=w223:dbl[], "Fase"=w219:dbl[])
                        n176 = Build Array (concatenate)(w219, w221) -> (w220:dbl[])
                        n177 = Build Array (concatenate)(w223, w221) -> (w222:dbl[])
                        n178 = Insert Into Array(array=w239, new element=w222) -> (w238:dbl[])  [unwired: 1 in]
                        n179 = Insert Into Array(array=w226, new element=w220) -> (w225:dbl[])  [unwired: 1 in]
                      }
                    }
                    n180 = local read "movXYZ"() -> (w161:T4)
                    n181 = local read "Y"() -> (w162:dbl)
                    n182 = Unbundle By Name(w161) -> ("Inicio x"=w160:dbl, "Inicio y"=w159:dbl)
                  }
                  n183 = local read "stop"() -> (w123:bool)
                  n184 = Build Array (concatenate)(w93, w94) -> (w95:dbl[][])
                  n185 = Build Array (concatenate)(w97, w98) -> (w99:dbl[][])
                  n186 = local read "X"() -> (w100:dbl)
                }
              }
              frame #4 {
                w572 = 0.0
                n187 = call "Movimiento nanometrico XYZ SIN CICLO.vi"("Movimiento en Z"=w572, "Movimiento en Y"=w572, "Movimiento en X"=w572) -> ()  [unwired: 3 in, 1 out]
                n188 = local write "X"(w572) -> ()
                n189 = local write "Y"(w572) -> ()
                n190 = local write "Z"(w572) -> ()
              }
              frame #5 {
                n191 = One Button Dialog(message="termino") -> ()  [unwired: 1 in, 1 out]
                n192 = local read "Nombre del  Archivo"() -> (w574:string)
                n193 = call "GuardadoTot.vi"("Atributos"=w573, "Fase"=w575, "Amplitud"=w576, "Nombre"=w574) -> ()  [unwired: 7 in, 1 out]
              }
            }
          }
        }
      }
      frame "visualizar" {
        n194 = case shown="True" "camara" {
          frame False {
          }
          frame True {
            n195 = call "camara.vi"("Nombre imagenes"="Nombre imagenes") -> ()  [unwired: 11 in]
          }
        }
        n196 = case shown="True" "Ajuste" {
          frame False {
          }
          frame True {
            n197 = call "AjusteLockIn.vi"() -> ()  [unwired: 12 in]
          }
        }
        n198 = case shown="True" "nanoREc" {
          frame False {
          }
          frame True {
            w581 = 0.0
            n199 = call "Movimiento nanometrico XYZ SIN CICLO.vi"("Movimiento en Z"=w581, "Movimiento en Y"=w581, "Movimiento en X"=w581) -> ()  [unwired: 3 in, 1 out]
          }
        }
      }
    }
  }
